vi "setCommandIdEvent.vi"(10 "CommandIdEvent":refnum<user-event>, 11 "UserEvents in":refnum<class "UserEvents.lvclass">) -> (3 "UserEvents out":refnum<class "UserEvents.lvclass">)   [LabVIEW 2016, in "UserEvents.lvclass"]
uses:
  UserEvents.lvclass
  Communicator/Topics/CommandId.ctl
  UserEvents.lvclass/UserEvents.ctl
  Communicator/M1M3Communicator.lvlib
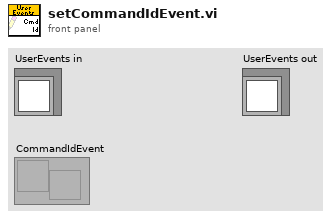
[diagram p1: front panel]
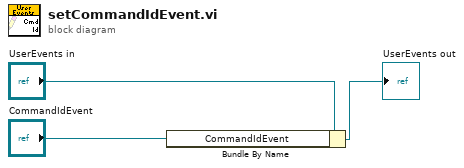
[diagram p0: block diagram]
diagram:
  n1 = Bundle By Name(cluster="UserEvents in", "CommandIdEvent"="CommandIdEvent") -> (→"UserEvents out":refnum<class "UserEvents.lvclass">)
